vi "Test Zentral Trigger PC.vi"() -> ()   [LabVIEW 2009]
uses:
  LV-BME Interface/ChnlSettings.ctl
  LV-BME Interface/BME_DG_TriggerSettings.ctl
  DG Classes/BME_DG_G05P2/SG05P2 Clock and Trigger Settings.ctl
  LV-BME Interface/ClockSource.ctl
  DG Classes/BME_DG_System/BME_DG_System.lvclass
  DG Classes/BME_DG_G05P2/BME_DG_G05P2.lvclass
  DG Classes/BME_DG_G05P2_Chnl/BME_DG_G05P2_Chnl.lvclass
  ChnlParam.ctl
  DG Classes/BME_DG_Base/BME_DG_Base.lvclass
  DG Classes/BME_DG_Chnl/BME_DG_Chnl.lvclass
panel:
  in  "Karten Parameter":T1[](array[typedef])=[{"Trigger"={"InputTerminated?"=TRUE, "InternalClockPeriode(µs)"=0.106293, "TriggerLevel"=-0.1001, "PresetValue"=0, "DivideBy"=4, "Clock Source"=3, "Gate Divider"=1, "PositiveGate?"=TRUE, "InternalTrigger?"=TRUE, "InternalArm?"=FALSE, "SWTrigger?"=FALSE, "RisingEdge?"=FALSE, "StopOnPreset?"=FALSE, "ResetWhenDone?"=FALSE, "TriggerEnabled?"=TRUE}, "ClockSource "=3, "V2 Trigger"={"Gate Type"=TRUE, "Synchronize Gate"=FALSE, "Force Trigger (µs)"=0.0, "MS Bus"=24}, " crystal oscillator"=6, "CardName"="Mira Sync"}, {"Trigger"={"InputTerminated?"=TRUE, "InternalClockPeriode(µs)"=99999.989371, "TriggerLevel"=1.401, "PresetValue"=0, "DivideBy"=1, "Clock Source"=3, "Gate Divider"=1, "PositiveGate?"=TRUE, "InternalTrigger?"=TRUE, "InternalArm?"=FALSE, "SWTrigger?"=FALSE, "RisingEdge?"=FALSE, "StopOnPreset?"=FALSE, "ResetWhenDone?"=FALSE, "TriggerEnabled?"=TRUE}, "ClockSource "=2, "V2 Trigger"={"Gate Type"=TRUE, "Synchronize Gate"=FALSE, "Force Trigger (µs)"=0.0, "MS Bus"=24}, " crystal oscillator"=1, "CardName"="FE PP"}, {"Trigger"={"InputTerminated?"=FALSE, "InternalClockPeriode(µs)"=0.0, "TriggerLevel"=1.25, "PresetValue"=0, "DivideBy"=1, "Clock Source"=3, "Gate Divider"=1, "PositiveGate?"=TRUE, "InternalTrigger?"=FALSE, "InternalArm?"=FALSE, "SWTrigger?"=FALSE, "RisingEdge?"=FALSE, "StopOnPreset?"=FALSE, "ResetWhenDone?"=FALSE, "TriggerEnabled?"=TRUE}, "ClockSource "=4, "V2 Trigger"={"Gate Type"=TRUE, "Synchronize Gate"=FALSE, "Force Trigger (µs)"=0.0, "MS Bus"=16}, " crystal oscillator"=8, "CardName"="A1 Haupt"}, {"Trigger"={"InputTerminated?"=TRUE, "InternalClockPeriode(µs)"=0.0, "TriggerLevel"=1.25, "PresetValue"=0, "DivideBy"=1, "Clock Source"=3, "Gate Divider"=1, "PositiveGate?"=TRUE, "InternalTrigger?"=FALSE, "InternalArm?"=FALSE, "SWTrigger?"=FALSE, "RisingEdge?"=FALSE, "StopOnPreset?"=FALSE, "ResetWhenDone?"=FALSE, "TriggerEnabled?"=TRUE}, "ClockSource "=4, "V2 Trigger"={"Gate Type"=TRUE, "Synchronize Gate"=FALSE, "Force Trigger (µs)"=0.0, "MS Bus"=16}, " crystal oscillator"=8, "CardName"="A1 Neben"}, {"Trigger"={"InputTerminated?"=FALSE, "InternalClockPeriode(µs)"=0.0, "TriggerLevel"=1.25, "PresetValue"=0, "DivideBy"=1, "Clock Source"=3, "Gate Divider"=1, "PositiveGate?"=TRUE, "InternalTrigger?"=TRUE, "InternalArm?"=FALSE, "SWTrigger?"=FALSE, "RisingEdge?"=FALSE, "StopOnPreset?"=FALSE, "ResetWhenDone?"=FALSE, "TriggerEnabled?"=TRUE}, "ClockSource "=4, "V2 Trigger"={"Gate Type"=TRUE, "Synchronize Gate"=FALSE, "Force Trigger (µs)"=0.0, "MS Bus"=16}, " crystal oscillator"=8, "CardName"="A2 Haupt"}, {"Trigger"={"InputTerminated?"=TRUE, "InternalClockPeriode(µs)"=0.0, "TriggerLevel"=1.25, "PresetValue"=0, "DivideBy"=1, "Clock Source"=3, "Gate Divider"=1, "PositiveGate?"=TRUE, "InternalTrigger?"=FALSE, "InternalArm?"=FALSE, "SWTrigger?"=FALSE, "RisingEdge?"=FALSE, "StopOnPreset?"=FALSE, "ResetWhenDone?"=FALSE, "TriggerEnabled?"=TRUE}, "ClockSource "=4, "V2 Trigger"={"Gate Type"=TRUE, "Synchronize Gate"=FALSE, "Force Trigger (µs)"=0.0, "MS Bus"=16}, " crystal oscillator"=1, "CardName"="A2 Neben"}, {"Trigger"={"InputTerminated?"=TRUE, "InternalClockPeriode(µs)"=0.0, "TriggerLevel"=1.25, "PresetValue"=0, "DivideBy"=1, "Clock Source"=3, "Gate Divider"=1, "PositiveGate?"=TRUE, "InternalTrigger?"=FALSE, "InternalArm?"=FALSE, "SWTrigger?"=FALSE, "RisingEdge?"=FALSE, "StopOnPreset?"=FALSE, "ResetWhenDone?"=FALSE, "TriggerEnabled?"=TRUE}, "ClockSource "=4, "V2 Trigger"={"Gate Type"=TRUE, "Synchronize Gate"=FALSE, "Force Trigger (µs)"=0.0, "MS Bus"=16}, " crystal oscillator"=1, "CardName"="A2 PP"}, {"Trigger"={"InputTerminated?"=TRUE, "InternalClockPeriode(µs)"=0.0, "TriggerLevel"=1.25, "PresetValue"=0, "DivideBy"=1, "Clock Source"=3, "Gate Divider"=1, "PositiveGate?"=TRUE, "InternalTrigger?"=FALSE, "InternalArm?"=FALSE, "SWTrigger?"=FALSE, "RisingEdge?"=FALSE, "StopOnPreset?"=FALSE, "ResetWhenDone?"=FALSE, "TriggerEnabled?"=TRUE}, "ClockSource "=4, "V2 Trigger"={"Gate Type"=TRUE, "Synchronize Gate"=FALSE, "Force Trigger (µs)"=0.0, "MS Bus"=16}, " crystal oscillator"=1, "CardName"="A2 PP, A2.5"}, {"Trigger"={"InputTerminated?"=TRUE, "InternalClockPeriode(µs)"=0.0, "TriggerLevel"=1.25, "PresetValue"=0, "DivideBy"=1, "Clock Source"=3, "Gate Divider"=1, "PositiveGate?"=TRUE, "InternalTrigger?"=FALSE, "InternalArm?"=FALSE, "SWTrigger?"=FALSE, "RisingEdge?"=FALSE, "StopOnPreset?"=FALSE, "ResetWhenDone?"=FALSE, "TriggerEnabled?"=TRUE}, "ClockSource "=4, "V2 Trigger"={"Gate Type"=TRUE, "Synchronize Gate"=FALSE, "Force Trigger (µs)"=0.0, "MS Bus"=16}, " crystal oscillator"=1, "CardName"="A3 Haupt"}, {"Trigger"={"InputTerminated?"=TRUE, "InternalClockPeriode(µs)"=0.0, "TriggerLevel"=1.25, "PresetValue"=0, "DivideBy"=1, "Clock Source"=3, "Gate Divider"=1, "PositiveGate?"=TRUE, "InternalTrigger?"=FALSE, "InternalArm?"=FALSE, "SWTrigger?"=FALSE, "RisingEdge?"=FALSE, "StopOnPreset?"=FALSE, "ResetWhenDone?"=FALSE, "TriggerEnabled?"=TRUE}, "ClockSource "=4, "V2 Trigger"={"Gate Type"=TRUE, "Synchronize Gate"=FALSE, "Force Trigger (µs)"=0.0, "MS Bus"=16}, " crystal oscillator"=1, "CardName"="A4 Haupt"}] {"V2 Trigger"."MS Bus" format="%04x" items=["Local Primary"=1, "Local Secondary"=2, "Local Force"=4, "Resynchronize"=8, "Master Primary"=16, "Master Secondary"=32, "Master Force"=64, "System Clock"=128, "Delay Clock"=256, "Inhibit Local"=512, "Start Local"=1024, "Start Bus"=2048, "Step Back Local"=4096, "Step Back Bus"=8192, "Enable From E"=65536, "Enable From F"=131072, "Enable From Bus"=262144]; "V2 Trigger"."Force Trigger (µs)" min=0.0 format="%.6f"; "ClockSource" items=["Internal Oscillator"=1, "External Trigger"=2, "Trigger & Oscillator"=3, "MasterSlave Bus"=4]; "Trigger"."Gate Divider" min=1 max=1000000; "Trigger"."Clock Source" items=["Internal Oscillator"=1, "External Trigger"=2, "Trigger & Oscillator"=3]; "Trigger"."InternalClockPeriode(µs)" format="%#_11g"}
  in  "Go Signal":u32(ring)=2048 items=["Local Primary"=1, "Local Secondary"=2, "Local Force"=4, "Resynchronize"=8, "Master Primary"=16, "Master Secondary"=32, "Master Force"=64, "System Clock"=128, "Delay Clock"=256, "Inhibit Local"=512, "Start Local"=1024, "Start Bus"=2048, "Step Back Local"=4096, "Step Back Bus"=8192, "From E"=65536, "From F"=131072, "From Bus"=262144]
  out "Problem Chnls out":string[](array[string])
  out "DelayFormulas":string[](array[string])
  in  "Reset Error":bool
  out "error out":errorcluster
  in  "Update Delay formula":bool=TRUE
  in  "DelayFormula":string="MasterSG02P2_ChnlT0 + 100"
  in  "Aknowledge interrupts":bool
  in  "stop 3":bool=TRUE
  in  "SetDelay":bool=TRUE
  in  "UpdateChnl":bool=TRUE
  in  "ChnlParameter":T5 {"ChnParam2write"."Delay (µs)" min=0.0 max=100000000.0 format="%.5f"}
  out "CountsRemains":i32
  out "TriggerCounters":i32[](array[numeric])
  out "Interrupts":u32[](array[numeric]) format="%b"
  out "RemainingTriggers":T6(array[cluster])=[[{"Time Stamp"=timestamp(3416308194.6875 s since 1904-01-01), "Numeric"=-64}, {"Time Stamp"=timestamp(3416308194.6875 s since 1904-01-01), "Numeric"=4}, {"Time Stamp"=timestamp(3416308194.6875 s since 1904-01-01), "Numeric"=-64}, {"Time Stamp"=timestamp(3416308194.6875 s since 1904-01-01), "Numeric"=-64}], [{"Time Stamp"=timestamp(3416308194.6875 s since 1904-01-01), "Numeric"=-64}, {"Time Stamp"=timestamp(3416308194.6875 s since 1904-01-01), "Numeric"=-64}, {"Time Stamp"=timestamp(3416308194.6875 s since 1904-01-01), "Numeric"=-64}, {"Time Stamp"=timestamp(3416308194.6875 s since 1904-01-01), "Numeric"=-64}], [{"Time Stamp"=timestamp(3416308194.6875 s since 1904-01-01), "Numeric"=-64}, {"Time Stamp"=timestamp(3416308194.6875 s since 1904-01-01), "Numeric"=-64}, {"Time Stamp"=timestamp(3416308194.6875 s since 1904-01-01), "Numeric"=-64}, {"Time Stamp"=timestamp(3416308194.6875 s since 1904-01-01), "Numeric"=-64}]] {"Time Stamp" format="%<%I:%M:%S%3u %p>T"}
  in  "stop 2":bool=TRUE
  in  "ReadStatus":bool=TRUE
  in  "Activate":bool
  in  "ResetModuloCounters":bool=TRUE
  in  "TriggerModulo":u32=4
  out "Modulo Settings":u32[](array[numeric])
  out "Chnls":T4[](array[typedef])=[{" Delay (µs)"=0.0, "On? (false)"=TRUE, "PositiveVoltage?"=TRUE, "50OhmTerminated? "=TRUE, "25OhmOutput?"=FALSE}, {" Delay (µs)"=0.0, "On? (false)"=TRUE, "PositiveVoltage?"=TRUE, "50OhmTerminated? "=TRUE, "25OhmOutput?"=FALSE}, {" Delay (µs)"=0.0, "On? (false)"=TRUE, "PositiveVoltage?"=TRUE, "50OhmTerminated? "=TRUE, "25OhmOutput?"=FALSE}] {"Delay (µs)" min=0.0 max=100000000.0 format="%.5f"}
  in  "Trigger Base":T2={"InputTerminated?"=FALSE, "InternalClockPeriode(µs)"=1000000.0, "TriggerLevel"=1.25, "PresetValue"=0, "DivideBy"=1, "Clock Source"=1, "Gate Divider"=1, "PositiveGate?"=TRUE, "InternalTrigger?"=FALSE, "InternalArm?"=FALSE, "SWTrigger?"=FALSE, "RisingEdge?"=FALSE, "StopOnPreset?"=FALSE, "ResetWhenDone?"=TRUE, "TriggerEnabled?"=TRUE} {"Gate Divider" min=1 max=1000000; "Clock Source" items=["Internal Oscillator"=1, "External Trigger"=2, "Trigger & Oscillator"=3]; "InternalClockPeriode(µs)" format="%#_11g"}
  in  "Selected Chnl":u16(ring) items=["MasterSG02P2_ChnlT0", "MasterSG02P2_ChnlA", "MasterSG02P2_ChnlB"]
  in  "Selected Card":u16(ring)=1 items=["MasterSG02P2", "Slave 1", "Slave 2", "MasterS08P1"]
  in  "STOP":bool=TRUE
  in  "ChnParam2write":T4={" Delay (µs)"=0.0, "On? (false)"=TRUE, "PositiveVoltage?"=TRUE, "50OhmTerminated? "=TRUE, "25OhmOutput?"=FALSE} {"Delay (µs)" min=0.0 max=100000000.0 format="%.5f"}
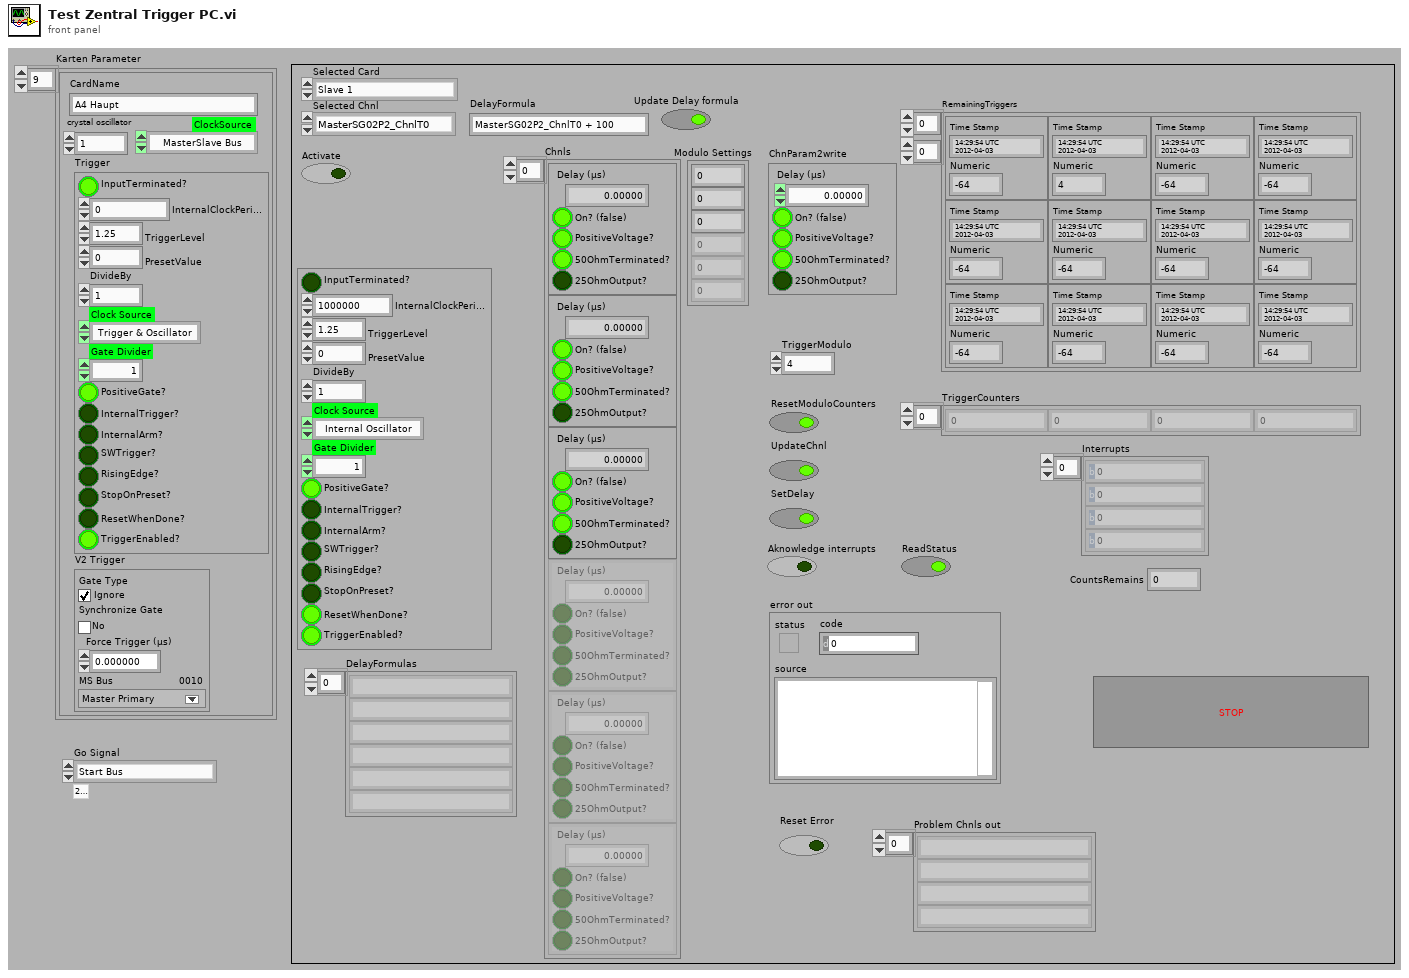
[diagram p1: front panel]
types:
  T1 = typedef "SG05P2 Clock and Trigger Settings.ctl" = cluster{"Trigger":T2, "ClockSource ":T3, "V2 Trigger":cluster{"Gate Type":bool, "Synchronize Gate":bool, "Force Trigger (µs)":dbl, "MS Bus":u32}, " crystal oscillator":u32, "CardName":string}
  T2 = typedef "BME_DG_TriggerSettings.ctl" = cluster{"InputTerminated?":bool, "InternalClockPeriode(µs)":dbl, "TriggerLevel":dbl, "PresetValue":i32, "DivideBy":i32, "Clock Source":u32, "Gate Divider":i32, "PositiveGate?":bool, "InternalTrigger?":bool, "InternalArm?":bool, "SWTrigger?":bool, "RisingEdge?":bool, "StopOnPreset?":bool, "ResetWhenDone?":bool, "TriggerEnabled?":bool}
  T3 = typedef "ClockSource.ctl" = i32
  T4 = typedef "ChnlSettings.ctl" = cluster{" Delay (µs)":dbl, "On? (false)":bool, "PositiveVoltage?":bool, "50OhmTerminated? ":bool, "25OhmOutput?":bool}
  T5 = cluster{"ChnlName":string, "ChnParam2write":T4, "TriggerModulo":u32}
  T6 = cluster{"Time Stamp":timestamp, "Numeric":i32}[][]
  T7 = typedef "ChnlParam.ctl" = cluster{"ChnlName":string, "DelayFormula":string, "OutputModulo":i32}
  T8 = cluster{"Gate Type":bool, "Synchronize Gate":bool, "Force Trigger (µs)":dbl, "MS Bus":u32}
  T9 = enum8{"Enabled", "Disabled", "Disabled and Grayed Out"}
  T10 = cluster{"ChnlName":string, "ChnParam2write":T4, "TriggerModulo":u32}[]
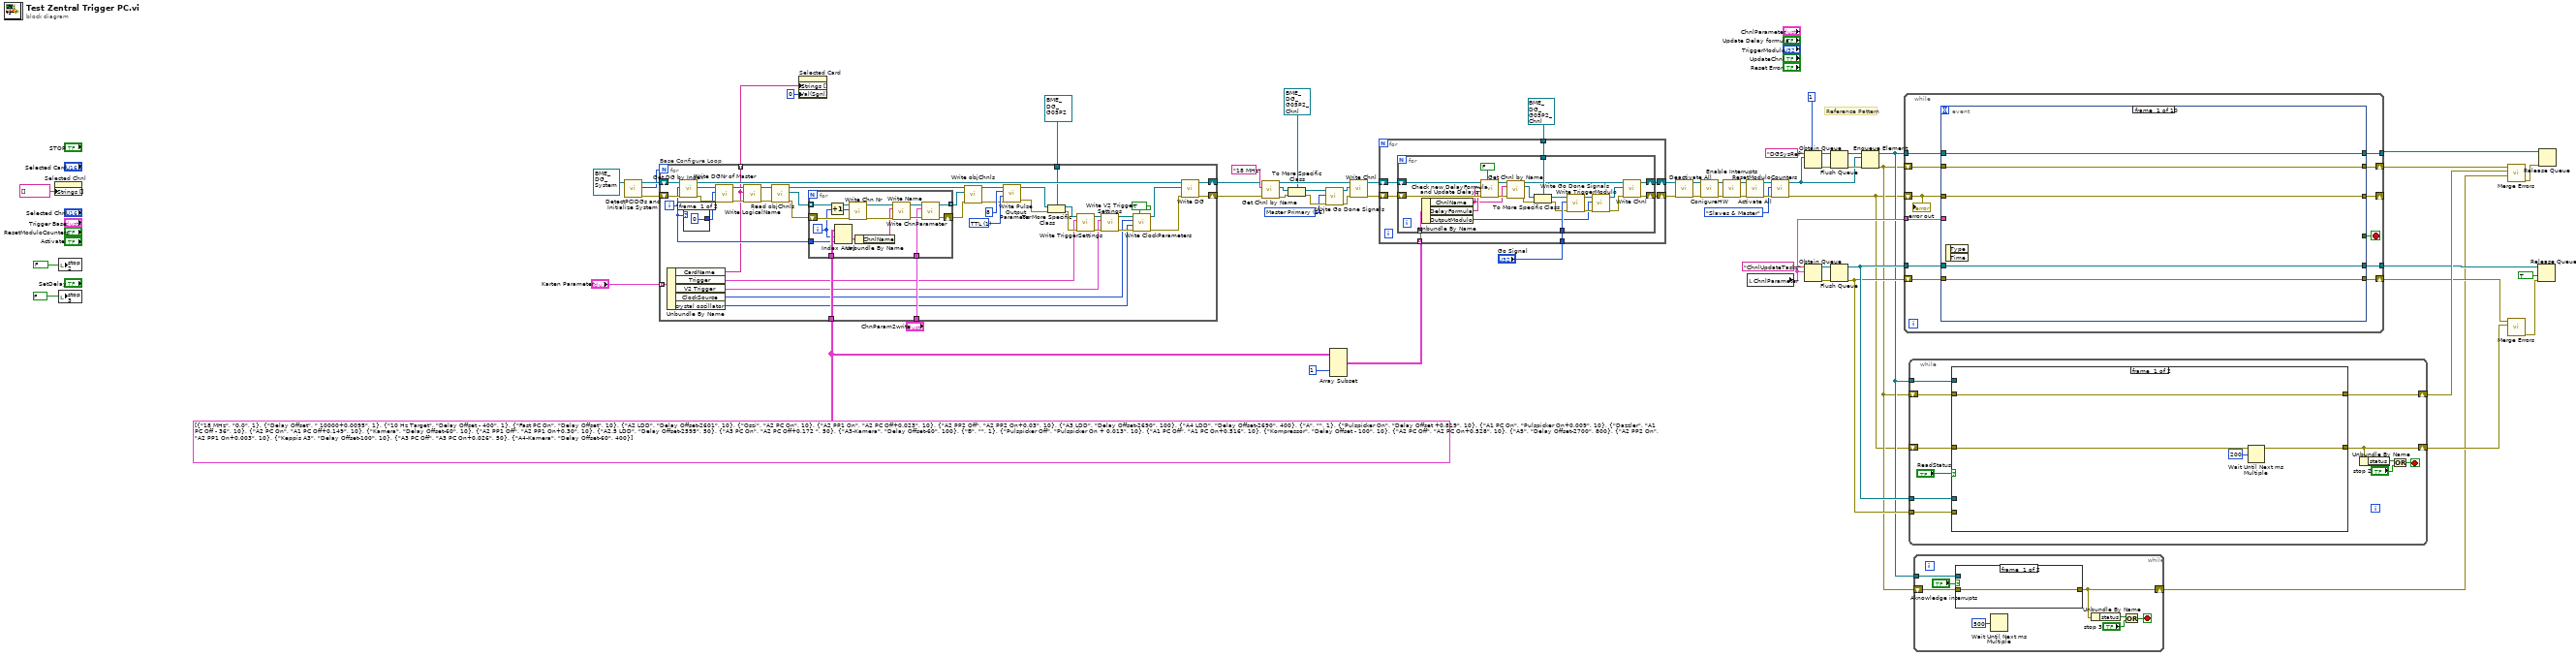
[diagram p0: block diagram]
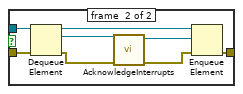
[diagram p2: hidden frame]
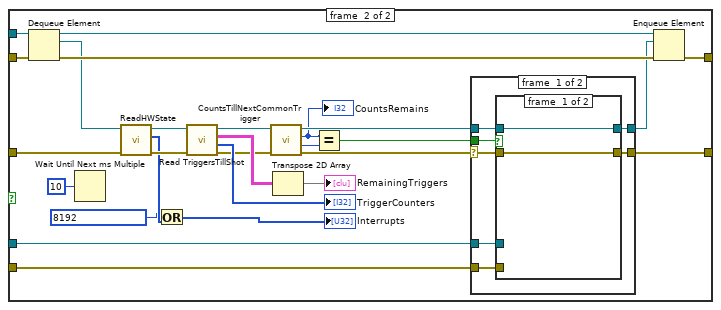
[diagram p3: hidden frame]
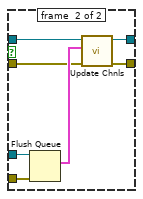
[diagram p4: hidden frame]
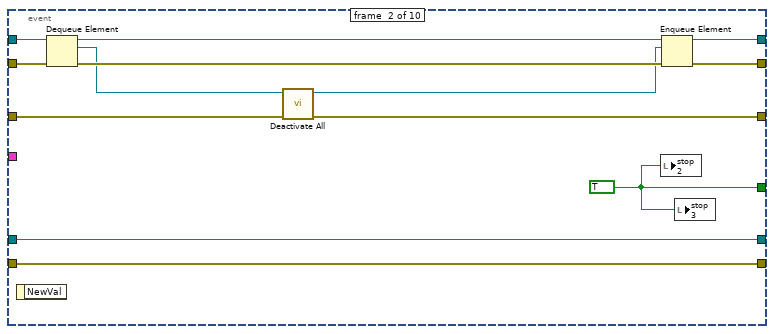
[diagram p6: hidden frame]
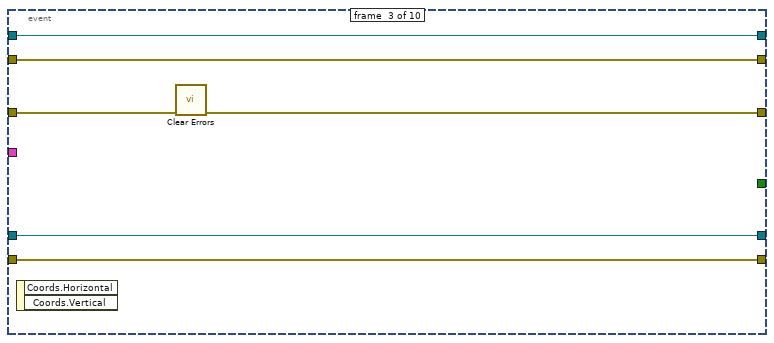
[diagram p7: hidden frame]
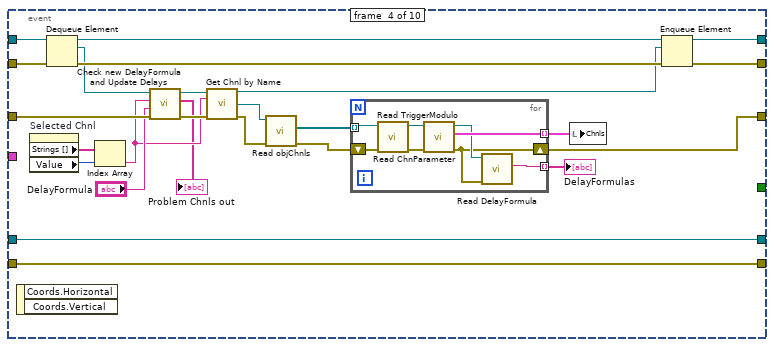
[diagram p8: hidden frame]
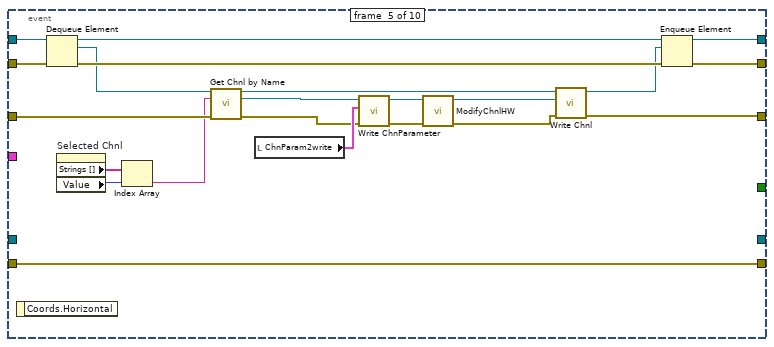
[diagram p9: hidden frame]
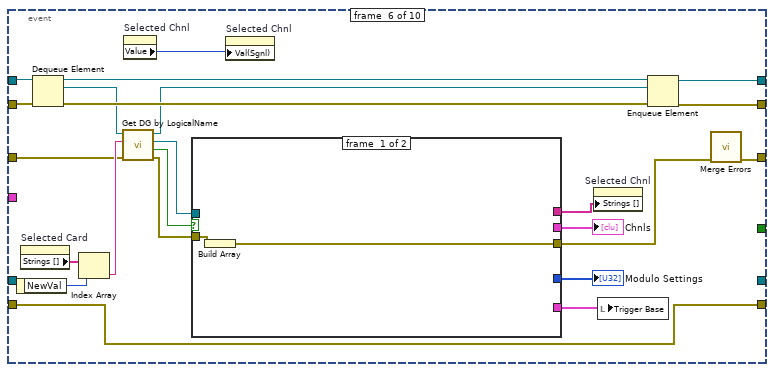
[diagram p10: hidden frame]
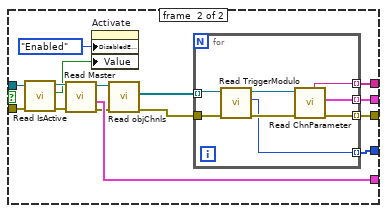
[diagram p11: hidden frame]
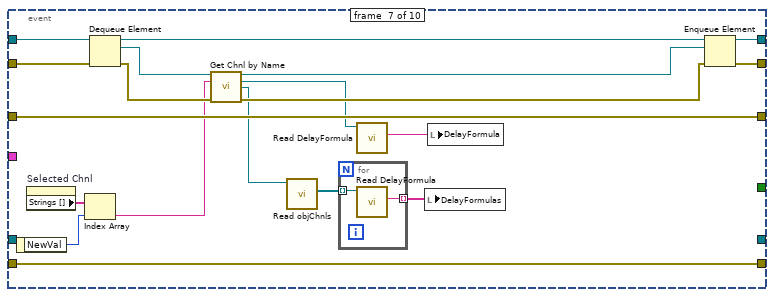
[diagram p12: hidden frame]
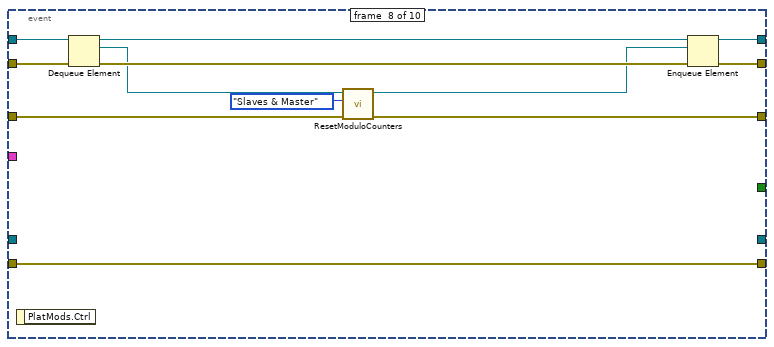
[diagram p13: hidden frame]
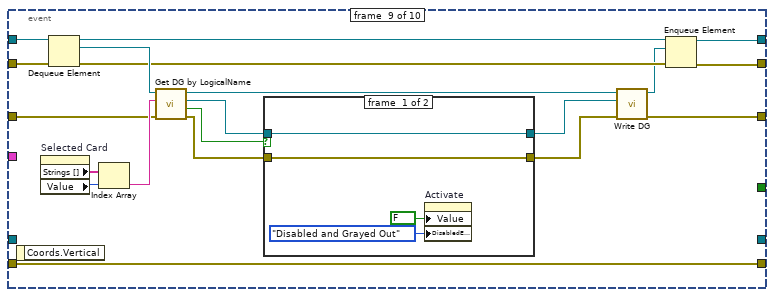
[diagram p14: hidden frame]
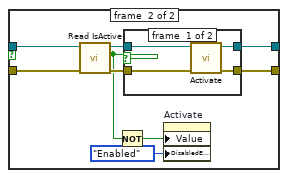
[diagram p15: hidden frame]
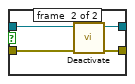
[diagram p16: hidden frame]
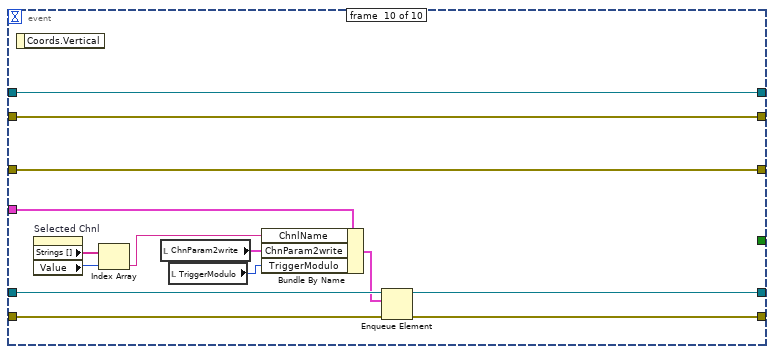
[diagram p17: hidden frame]
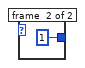
[diagram p18: hidden frame]
diagram:
  w10 = T7[][] [[{"ChnlName"="18 MHz", "DelayFormula"="0.0", "OutputModulo"=1}, {"ChnlName"="Delay Offset", "DelayFormula"=" 10000+0.0095", "OutputModulo"=1}, {"ChnlName"="10 Hz Target", "DelayFormula"="Delay Offset - 400", "OutputModulo"=1}, {"ChnlName"="Fast PC On", "DelayFormula"="Delay Offset", "OutputModulo"=10}, {"ChnlName"="A2 LDD", "DelayFormula"="Delay Offset-2601", "OutputModulo"=10}, {"ChnlName"="Oszi", "DelayFormula"="A2 PC On", "OutputModulo"=10}, {"ChnlName"="A2 PP1 On", "DelayFormula"="A2 PC Off+0.023", "OutputModulo"=10}, {"ChnlName"="A2 PP2 Off", "DelayFormula"="A2 PP2 On+0.03", "OutputModulo"=10}, {"ChnlName"="A3 LDD", "DelayFormula"="Delay Offset-2690", "OutputModulo"=100}, {"ChnlName"="A4 LDD", "DelayFormula"="Delay Offset-2690", "OutputModulo"=400}], [{"ChnlName"="A", "DelayFormula"="", "OutputModulo"=1}, {"ChnlName"="Pulspicker On", "DelayFormula"="Delay Offset +0.819", "OutputModulo"=10}, {"ChnlName"="A1 PC On", "DelayFormula"="Pulspicker On+0.009", "OutputModulo"=10}, {"ChnlName"="Dazzler", "DelayFormula"="A1 PC Off - 36", "OutputModulo"=10}, {"ChnlName"="A2 PC On", "DelayFormula"="A1 PC Off+0.149", "OutputModulo"=10}, {"ChnlName"="Kamera", "DelayFormula"="Delay Offset-60", "OutputModulo"=10}, {"ChnlName"="A2 PP1 Off", "DelayFormula"="A2 PP1 On+0.30", "OutputModulo"=10}, {"ChnlName"="A2.5 LDD", "DelayFormula"="Delay Offset-2595", "OutputModulo"=50}, {"ChnlName"="A3 PC On", "DelayFormula"="A2 PC Off+0.172 ", "OutputModulo"=50}, {"ChnlName"="A3-Kamera", "DelayFormula"="Delay Offset-60", "OutputModulo"=100}], [{"ChnlName"="B", "DelayFormula"="", "OutputModulo"=1}, {"ChnlName"="Pulspicker Off", "DelayFormula"="Pulspicker On + 0.013", "OutputModulo"=10}, {"ChnlName"="A1 PC Off", "DelayFormula"="A1 PC On+0.516", "OutputModulo"=10}, {"ChnlName"="Kompressor", "DelayFormula"="Delay Offset - 100", "OutputModulo"=10}, {"ChnlName"="A2 PC Off", "DelayFormula"="A2 PC On+0.528", "OutputModulo"=10}, {"ChnlName"="A5", "DelayFormula"="Delay Offset-2700", "OutputModulo"=800}, {"ChnlName"="A2 PP2 On", "DelayFormula"="A2 PP1 On+0.003", "OutputModulo"=10}, {"ChnlName"="Keppis A3", "DelayFormula"="Delay Offset-100", "OutputModulo"=10}, {"ChnlName"="A3 PC Off", "DelayFormula"="A3 PC On+0.026", "OutputModulo"=50}, {"ChnlName"="A4-Kamera", "DelayFormula"="Delay Offset-60", "OutputModulo"=400}]] ("ChnlParam 2")
  w14 = u32 16 items=["Local Primary"=1, "Local Secondary"=2, "Local Force"=4, "Resynchronize"=8, "Master Primary"=16, "Master Secondary"=32, "Master Force"=64, "System Clock"=128, "Delay Clock"=256, "Inhibit Local"=512, "Start Local"=1024, "Start Bus"=2048, "Step Back Local"=4096, "Step Back Bus"=8192, "From E"=65536, "From F"=131072, "From Bus"=262144] ("Go Signal")
  # "Reference Pattern"
  n1 = property on="Selected Chnl" class="Ring (strict)"("Strings []"=string[] []) -> ()  [unwired: 2 in, 2 out]
  n2 = local write "stop 2"(FALSE ("stop 2")) -> ()
  n3 = local write "stop 3"(FALSE ("stop 3")) -> ()
  n4 = call "DetectPCIDGs and Initialize System.vi"("BME_DG_System in"=refnum<class "BME_DG_System.lvclass"> refnum ("BME_DG_System.lvclass")) -> ("error out"=w66:errorcluster, "NumberOfCards"=w65:i32, "BME_DG_System out"=w67:refnum<class "BME_DG_System.lvclass">)  [unwired: 8 in]
  n5 = for "Base Configure Loop" {
    N: w65 -> [_]
    shift-right: [w107] -> w5
    shift-left: w67 -> [w110]
    shift-right: [w106] -> w4
    shift-left: w66 -> [w109]
    tunnel: "ChnParam2write" -> [w103]
    tunnel: w10 -> [w99]
    tunnel: [w85] -> w39 mode=indexing
    tunnel: "Karten Parameter" -> [w86] mode=indexing
    tunnel: refnum<class "BME_DG_G05P2.lvclass"> refnum ("BME_DG_G05P2.lvclass") -> [w78]
    i -> [w92]
    w88 = u32 1 items=["TTL"=1, "NIM"=2, "ECL"=3] ("Pulse Output Level")
    n6 = Unbundle By Name(w86) -> ("CardName"=w85:string, "Trigger"=w72:T2, "V2 Trigger"=w71:T8, "ClockSource"=w69:T3, "crystal oscillator"=w70:u32)
    n7 = call "Get DG by Index.vi"("error in (no error)"=w109, "index"=w92, "BME_DG_System in"=w110) -> ("error out"=w93:errorcluster, "BME_DG_Base.lvclass"=w96:refnum<class "BME_DG_Base.lvclass">, "BME_DG_System out"=w108:refnum<class "BME_DG_System.lvclass">)  [unwired: 6 in]
    n8 = case shown="1, Default" w92 {
      tunnel: [0 1] -> w91
      frame #0 {
      }
      frame #1 {
      }
    }
    n9 = call-dynamic "Write DGNr of Master.vi"("error in (no error)"=w93, "DGNr of Master"=w91, "BME_DG_Base in"=w96) -> ("error out"=w94:errorcluster, "BME_DG_Base out"=w95:refnum<class "BME_DG_Base.lvclass">)  [unwired: 7 in]
    n10 = call "Write LogicalName.vi"("error in (no error)"=w94, "LogicalName"=w85, "BME_DG_Base in"=w95) -> ("error out"=w97:errorcluster, "BME_DG_Base out"=w98:refnum<class "BME_DG_Base.lvclass">)  [unwired: 7 in]
    n11 = call-dynamic "Read objChnls.vi"("error in (no error)"=w97, "BME_DG_Base in"=w98) -> ("error out"=w104:errorcluster, "objChnls"=w105:refnum<class "BME_DG_Chnl.lvclass">[], "BME_DG_Base out"=w101:refnum<class "BME_DG_Base.lvclass">)  [unwired: 6 in, 1 out]
    n12 = for {
      tunnel: w105 -> [w124] mode=indexing
      shift-right: [w116] -> w100
      shift-left: w104 -> [w122]
      tunnel: w103 -> [w125]
      tunnel: [w117] -> w102 mode=indexing
      tunnel: w99 -> [w119]
      tunnel: w92 -> [w114]
      i -> [w115]
      n13 = Increment(x=w115) -> (x+1=w120:i32)
      n14 = Index Array(array=w119, index (row)=w115, index (col)=w114) -> (element=w118:T7)
      n15 = call-dynamic "Write Chn Nr.vi"("error in (no error)"=w122, "Chn Nr"=w120, "BME_DG_Chnl in"=w124) -> ("error out"=w121:errorcluster, "BME_DG_Chnl out"=w123:refnum<class "BME_DG_Chnl.lvclass">)  [unwired: 7 in]
      n16 = Unbundle By Name(w118) -> ("ChnlName"=w113:string)
      n17 = call-dynamic "Write Name.vi"("error in (no error)"=w121, "Name"=w113, "BME_DG_Chnl in"=w123) -> ("error out"=w126:errorcluster, "BME_DG_Chnl out"=w127:refnum<class "BME_DG_Chnl.lvclass">)  [unwired: 7 in]
      n18 = call-dynamic "Write ChnParameter.vi"("error in (no error)"=w126, "ChnParemater"=w125, "BME_DG_Chnl in"=w127) -> ("error out"=w116:errorcluster, "BME_DG_Chnl out"=w117:refnum<class "BME_DG_Chnl.lvclass">)  [unwired: 7 in]
    }
    n19 = call-dynamic "Write objChnls.vi"("error in (no error)"=w100, "objChnls"=w102, "BME_DG_Base in"=w101) -> ("error out"=w87:errorcluster, "BME_DG_Base out"=w90:refnum<class "BME_DG_Base.lvclass">)  [unwired: 7 in]
    n20 = call-dynamic "Write Pulse Output Parameter.vi"("error in (no error)"=w87, "Pulse Output Level"=w88, "Pulse Width"=u32 8, "BME_DG_Base in"=w90) -> ("error out"=w75:errorcluster, "BME_DG_Base out"=w77:refnum<class "BME_DG_Base.lvclass">)  [unwired: 6 in]
    n21 = To More Specific Class(target class=w78, reference=w77, error in=w75) -> (specific class reference=w79:refnum<class "BME_DG_G05P2.lvclass">, error out=w80:errorcluster)
    n22 = call-dynamic "Write TriggerSettings.vi"("error in (no error)"=w80, "Trigger Settings"=w72, "BME_DG_Base in"=w79) -> ("error out"=w83:errorcluster, "BME_DG_Base out"=w81:refnum<class "BME_DG_G05P2.lvclass">)  [unwired: 7 in]
    n23 = call-dynamic "Write V2 Trigger Settings.vi"("error in (no error)"=w83, "V2 Trigger Settings"=w71, "BME_DG_G05 in"=w81) -> ("error out"=w84:errorcluster, "BME_DG_G05 out"=w82:refnum<class "BME_DG_G05P2.lvclass">)  [unwired: 7 in]
    n24 = call-dynamic "Write ClockParameters.vi"("ClockEnable"=TRUE, "error in (no error)"=w84, "PrescalerCrystalOscilator"=w70, "ClockSource"=w69, "BME_DG_Base in"=w82) -> ("error out"=w74:errorcluster, "BME_DG_Base out"=w76:refnum<class "BME_DG_G05P2.lvclass">)  [unwired: 5 in]
    n25 = call "Write DG.vi"("error in (no error)"=w74, "BME_DG_Base"=w76, "BME_DG_System in"=w108) -> ("error out"=w106:errorcluster, "BME_DG_System out"=w107:refnum<class "BME_DG_System.lvclass">)  [unwired: 7 in]
  }
  n26 = property on="Selected Card" class="Ring (strict)"("Strings []"=w39, "Val(Sgnl)"=u16 0 ("Value (Signaling)")) -> ()  [unwired: 2 in, 2 out]
  n27 = call "Get Chnl by Name.vi"("BME_DG_System in"=w5, "Chnl Name"="18 MHz", "error in (no error)"=w4) -> ("BME_DG_System out"=w22:refnum<class "BME_DG_System.lvclass">, "BME_DG_Chnl"=w21:refnum<class "BME_DG_Chnl.lvclass">, "error out"=w18:errorcluster)  [unwired: 7 in, 3 out]
  n28 = To More Specific Class(target class=refnum<class "BME_DG_G05P2_Chnl.lvclass"> refnum ("BME_DG_G05P2_Chnl.lvclass"), reference=w21, error in=w18) -> (specific class reference=w20:refnum<class "BME_DG_G05P2_Chnl.lvclass">, error out=w17:errorcluster)
  n29 = call-dynamic "Write Go Done Signals.vi"("error in (no error)"=w17, "Go Signal"=w14, "BME_DG_G05P2_Chnl in"=w20) -> ("error out"=w16:errorcluster, "BME_DG_G05P2_Chnl out"=w15:refnum<class "BME_DG_G05P2_Chnl.lvclass">)  [unwired: 7 in]
  n30 = Array Subset(array=w10, index (col)=1 ("index")) -> (w11:T7[][])  [unwired: 3 in]
  n31 = call "Write Chnl.vi"("error in (no error)"=w16, "BME_DG_Chnl.lvclass"=w15, "BME_DG_System in"=w22) -> ("error out"=w1:errorcluster, "BME_DG_System out"=w2:refnum<class "BME_DG_System.lvclass">)  [unwired: 7 in]
  n32 = for {
    shift-right: [w133] -> w13
    shift-left: w2 -> [w134]
    shift-right: [w131] -> w12
    shift-left: w1 -> [w132]
    tunnel: w11 -> [w130] mode=indexing
    tunnel: refnum<class "BME_DG_G05P2_Chnl.lvclass"> refnum ("BME_DG_G05P2_Chnl.lvclass") -> [w129]
    tunnel: "Go Signal" -> [w128]
    n33 = for {
      shift-right: [w139] -> w133
      shift-left: w134 -> [w156]
      shift-right: [w138] -> w131
      shift-left: w132 -> [w155]
      tunnel: w130 -> [w153] mode=indexing
      tunnel: w129 -> [w147]
      tunnel: w128 -> [w145]
      n34 = Unbundle By Name(w153) -> ("ChnlName"=w149:string, "DelayFormula"=w152:string, "OutputModulo"=w140:i32)
      n35 = call "Check new DelayFormula and Update Delays.vi"("Update HW"=FALSE, "error in (no error)"=w155, "Delay Formula"=w152, "ChnlName"=w149, "BME_DG_System in"=w156) -> ("error out"=w150:errorcluster, "BME_DG_System out"=w151:refnum<class "BME_DG_System.lvclass">)  [unwired: 4 in, 1 out]
      n36 = call "Get Chnl by Name.vi"("BME_DG_System in"=w151, "Chnl Name"=w149, "error in (no error)"=w150) -> ("BME_DG_System out"=w137:refnum<class "BME_DG_System.lvclass">, "BME_DG_Chnl"=w146:refnum<class "BME_DG_Chnl.lvclass">, "error out"=w144:errorcluster)  [unwired: 7 in, 3 out]
      n37 = To More Specific Class(target class=w147, reference=w146, error in=w144) -> (specific class reference=w148:refnum<class "BME_DG_G05P2_Chnl.lvclass">, error out=w143:errorcluster)
      n38 = call-dynamic "Write Go Done Signals.vi"("error in (no error)"=w143, "Go Signal"=w145, "BME_DG_G05P2_Chnl in"=w148) -> ("error out"=w141:errorcluster, "BME_DG_G05P2_Chnl out"=w142:refnum<class "BME_DG_G05P2_Chnl.lvclass">)  [unwired: 7 in]
      n39 = call-dynamic "Write TriggerModulo.vi"("error in (no error)"=w141, "TriggerModulo"=w140, "BME_DG_G05_Chnl in"=w142) -> ("error out"=w136:errorcluster, "BME_DG_G05_Chnl out"=w135:refnum<class "BME_DG_G05P2_Chnl.lvclass">)  [unwired: 7 in]
      n40 = call "Write Chnl.vi"("error in (no error)"=w136, "BME_DG_Chnl.lvclass"=w135, "BME_DG_System in"=w137) -> ("error out"=w138:errorcluster, "BME_DG_System out"=w139:refnum<class "BME_DG_System.lvclass">)  [unwired: 7 in]
    }
  }
  n41 = call "Deactivate All.vi"("error in (no error)"=w12, "BME_DG_System in"=w13) -> ("error out"=w37:errorcluster, "BME_DG_System out"=w38:refnum<class "BME_DG_System.lvclass">)  [unwired: 8 in]
  n42 = call "ConigureHW.vi"("error in (no error)"=w37, "BME_DG_System in"=w38) -> ("error out"=w35:errorcluster, "BME_DG_System out"=w36:refnum<class "BME_DG_System.lvclass">)  [unwired: 8 in]
  n43 = call "Enable Interrupts.vi"("error in (no error)"=w35, "BME_DG_System in"=w36) -> ("error out"=w29:errorcluster, "BME_DG_System out"=w30:refnum<class "BME_DG_System.lvclass">)  [unwired: 8 in]
  n44 = call "Activate All.vi"("error in (no error)"=w29, "BME_DG_System in"=w30) -> ("error out"=w26:errorcluster, "BME_DG_System out"=w28:refnum<class "BME_DG_System.lvclass">)  [unwired: 8 in]
  n45 = local read "ChnlParameter"() -> (w47:T5)
  n46 = call "ResetModuloCounters.vi"("error in (no error)"=w26, "Enum"=enum16{"Slaves only", "Slaves & Master"}."Slaves & Master", "BME_DG_System in"=w28) -> ("error out"=w25:errorcluster, "BME_DG_System out"=w27:refnum<class "BME_DG_System.lvclass">)  [unwired: 7 in]
  n47 = Obtain Queue(max queue size (-1, unlimited)=1, name (unnamed)="DGSysRef", element data type=w27) -> (queue out=w55:refnum<queue>, error out=w53:errorcluster)  [unwired: 2 in, 1 out]
  n48 = Obtain Queue(name (unnamed)="ChnlUpdateTasks", element data type=w47) -> (queue out=w48:refnum<queue>, error out=w49:errorcluster)  [unwired: 3 in, 1 out]
  n49 = Flush Queue(queue=w55, error in (no error)=w53) -> (queue out=w54:refnum<queue>, error out=w52:errorcluster)  [unwired: 1 out]
  n50 = Flush Queue(queue=w48, error in (no error)=w49) -> (queue out=w44:refnum<queue>, error out=w43:errorcluster)  [unwired: 1 out]
  n51 = Enqueue Element(queue=w54, element=w27, error in (no error)=w52) -> (queue out=w34:refnum<queue>, error out=w33:errorcluster)  [unwired: 1 in, 1 out]
  n52 = while {
    shift-right: [w164] -> _
    shift-left: w25 -> [w166]
    shift-right: [w162] -> w58
    shift-left: w33 -> [w163]
    tunnel: w34 -> [w167]
    tunnel: [w165] -> w60
    tunnel: w44 -> [w161]
    tunnel: w47 -> [w160]
    tunnel: [w158] -> w46
    shift-right: [w157] -> w42
    shift-left: w43 -> [w159]
    stop <- w168 stop-if-true
    n53 = event shown="[3] \"Update Delay formula\": Mouse Down" {
      selector: _ -> [_ _ _ _ _ _ _ _ _ _]
      dyn-events: _ -> [_ _ _ _ _ _ _ _ _ _]
      timeout: _ -> [_ _ _ _ _ _ _ _ _ _]
      tunnel: [_ w174 _ _ _ _ _ _ _ _] -> w168
      tunnel: w167 -> [w173 w183 w191 w216 w246 w258 w309 w328 w337 w383]
      tunnel: w166 -> [w172 w186 w192 w208 w237 w267 w314 w318 w345 w382]
      tunnel: [w173 w179 w191 w212 w242 w256 w307 w323 w331 w383] -> w165
      tunnel: [w172 w185 w187 w196 w226 w251 w314 w319 w338 w382] -> w164
      tunnel: w163 -> [w171 w182 w190 w215 w245 w257 w308 w326 w336 w379]
      tunnel: [w171 w180 w190 w213 w243 w255 w306 w324 w330 w379] -> w162
      tunnel: w161 -> [w170 w176 w189 w211 _ _ _ _ _ w374]
      tunnel: w160 -> [_ _ _ _ _ _ _ _ _ w378]
      tunnel: w159 -> [w169 w175 w188 w210 w241 w249 w313 w322 w329 w372]
      tunnel: [w170 w176 w189 w211 _ _ _ _ _ w371] -> w158
      tunnel: [w169 w175 w188 w210 w241 w249 w313 w322 w329 w370] -> w157
      event #0 {
        n54 = event-data() -> ()  [unwired: 1 in, 2 out]
      }
      event #1 {
        w174 = TRUE
        n55 = event-data() -> ()  [unwired: 1 in, 1 out]
        n56 = Dequeue Element(queue=w183, error in (no error)=w182) -> (queue out=w184:refnum<queue>, element=w177:refnum<class "BME_DG_System.lvclass">, error out=w181:errorcluster)  [unwired: 1 in, 1 out]
        n57 = call "Deactivate All.vi"("error in (no error)"=w186, "BME_DG_System in"=w177) -> ("error out"=w185:errorcluster, "BME_DG_System out"=w178:refnum<class "BME_DG_System.lvclass">)  [unwired: 8 in]
        n58 = local write "stop 2"(w174) -> ()
        n59 = Enqueue Element(queue=w184, element=w178, error in (no error)=w181) -> (queue out=w179:refnum<queue>, error out=w180:errorcluster)  [unwired: 1 in, 1 out]
        n60 = local write "stop 3"(w174) -> ()
      }
      event #2 {
        n61 = event-data() -> ()  [unwired: 1 in, 2 out]
        n62 = call <vilib>:"Clear Errors.vi"("error in (no error)"=w192) -> ("error out"=w187:errorcluster)  [unwired: 6 in]
      }
      event #3 {
        n63 = event-data() -> ()  [unwired: 1 in, 2 out]
        n64 = property on="Selected Chnl" class="Ring (strict)"() -> ("Strings []"=w206:string[], "Value"=w207:u16)  [unwired: 2 in, 2 out]
        n65 = Dequeue Element(queue=w216, error in (no error)=w215) -> (queue out=w217:refnum<queue>, element=w209:refnum<class "BME_DG_System.lvclass">, error out=w214:errorcluster)  [unwired: 1 in, 1 out]
        n66 = Index Array(array=w206, index=w207) -> (element=w195:string)
        n67 = call "Check new DelayFormula and Update Delays.vi"("error in (no error)"=w208, "Delay Formula"="DelayFormula", "ChnlName"=w195, "BME_DG_System in"=w209) -> ("error out"=w198:errorcluster, "Problem Chnls out"=→"Problem Chnls out":string[], "BME_DG_System out"=w200:refnum<class "BME_DG_System.lvclass">)  [unwired: 5 in]
        n68 = call "Get Chnl by Name.vi"("BME_DG_System in"=w200, "Chnl Name"=w195, "error in (no error)"=w198) -> ("BME_DG_System out"=w199:refnum<class "BME_DG_System.lvclass">, "Owner DG"=w201:refnum<class "BME_DG_Base.lvclass">, "error out"=w197:errorcluster)  [unwired: 7 in, 3 out]
        n69 = call-dynamic "Read objChnls.vi"("error in (no error)"=w197, "BME_DG_Base in"=w201) -> ("error out"=w202:errorcluster, "objChnls"=w204:refnum<class "BME_DG_Chnl.lvclass">[])  [unwired: 6 in, 2 out]
        n70 = for {
          tunnel: w204 -> [w224] mode=indexing
          tunnel: [w225] -> w203 mode=indexing
          shift-right: [w219] -> w196
          shift-left: w202 -> [w222]
          tunnel: [w218] -> w194 mode=indexing
          n71 = call-dynamic "Read TriggerModulo.vi"("error in (no error)"=w222, "BME_DG_Chnl in"=w224) -> ("error out"=w221:errorcluster, "BME_DG_Chnl out"=w223:refnum<class "BME_DG_Chnl.lvclass">)  [unwired: 7 in, 1 out]
          n72 = call-dynamic "Read ChnParameter.vi"("error in (no error)"=w221, "BME_DG_Chnl in"=w223) -> ("error out"=w219:errorcluster, "ChnParemater"=w225:T4, "BME_DG_Chnl out"=w220:refnum<class "BME_DG_Chnl.lvclass">)  [unwired: 4 in, 3 out]
          n73 = call-dynamic "Read DelayFormula.vi"("error in (no error)"=w219, "BME_DG_Chnl in"=w220) -> ("DelayFormula"=w218:string)  [unwired: 7 in, 2 out]
        }
        "DelayFormulas" <- w194
        n74 = local write "Chnls"(w203) -> ()
        n75 = Enqueue Element(queue=w217, element=w199, error in (no error)=w214) -> (queue out=w212:refnum<queue>, error out=w213:errorcluster)  [unwired: 1 in, 1 out]
      }
      event #4 {
        n76 = event-data() -> ()  [unwired: 1 in, 1 out]
        n77 = Dequeue Element(queue=w246, error in (no error)=w245) -> (queue out=w247:refnum<queue>, element=w238:refnum<class "BME_DG_System.lvclass">, error out=w244:errorcluster)  [unwired: 1 in, 1 out]
        n78 = property on="Selected Chnl" class="Ring (strict)"() -> ("Strings []"=w239:string[], "Value"=w240:u16)  [unwired: 2 in, 2 out]
        n79 = Index Array(array=w239, index=w240) -> (element=w236:string)
        n80 = call "Get Chnl by Name.vi"("BME_DG_System in"=w238, "Chnl Name"=w236, "error in (no error)"=w237) -> ("BME_DG_System out"=w232:refnum<class "BME_DG_System.lvclass">, "BME_DG_Chnl"=w235:refnum<class "BME_DG_Chnl.lvclass">, "error out"=w233:errorcluster)  [unwired: 7 in, 3 out]
        n81 = local read "ChnParam2write"() -> (w234:T4)
        n82 = call-dynamic "Write ChnParameter.vi"("error in (no error)"=w233, "ChnParemater"=w234, "BME_DG_Chnl in"=w235) -> ("error out"=w229:errorcluster, "BME_DG_Chnl out"=w230:refnum<class "BME_DG_Chnl.lvclass">)  [unwired: 7 in]
        n83 = call-dynamic "ModifyChnlHW.vi"("error in (no error)"=w229, "BME_DG_Chnl in"=w230) -> ("error out"=w227:errorcluster, "BME_DG_Chnl out"=w228:refnum<class "BME_DG_Chnl.lvclass">)  [unwired: 8 in]
        n84 = call "Write Chnl.vi"("error in (no error)"=w227, "BME_DG_Chnl.lvclass"=w228, "BME_DG_System in"=w232) -> ("error out"=w226:errorcluster, "BME_DG_System out"=w231:refnum<class "BME_DG_System.lvclass">)  [unwired: 7 in]
        n85 = Enqueue Element(queue=w247, element=w231, error in (no error)=w244) -> (queue out=w242:refnum<queue>, error out=w243:errorcluster)  [unwired: 1 in, 1 out]
      }
      event #5 {
        n86 = event-data() -> ("NewVal"=w269:u16)  [unwired: 1 in]
        n87 = property on="Selected Card" class="Ring (strict)"() -> ("Strings []"=w270:string[])  [unwired: 2 in, 2 out]
        n88 = Dequeue Element(queue=w258, error in (no error)=w257) -> (queue out=w259:refnum<queue>, element=w254:refnum<class "BME_DG_System.lvclass">, error out=w260:errorcluster)  [unwired: 1 in, 1 out]
        n89 = Index Array(array=w270, index=w269) -> (element=w268:string)
        n90 = call "Get DG by LogicalName.vi"("error in (no error)"=w267, "LogicalName"=w268, "BME_DG_System in"=w254) -> ("error out"=w252:errorcluster, "found?"=w266:bool, "BME_DG_Base.lvclass"=w265:refnum<class "BME_DG_Base.lvclass">, "BME_DG_System out"=w253:refnum<class "BME_DG_System.lvclass">)  [unwired: 5 in]
        n91 = property on="Selected Chnl" class="Ring (strict)"() -> ("Value"=w248:u16)  [unwired: 2 in, 2 out]
        n92 = case shown="True" w266 {
          tunnel: w265 -> [_ w280]
          tunnel: [_ w287] -> w264
          tunnel: [_ w286] -> w262
          tunnel: [_ w285] -> w263
          tunnel: [_ w281] -> w261
          tunnel: w252 -> [w272 w277]
          tunnel: [w271 w275] -> w250
          frame #0 {
            n93 = Build Array(w272) -> (w271:errorcluster[])
          }
          frame #1 {
            n94 = call-dynamic "Read IsActive.vi"("error in (no error)"=w277, "BME_DG_Base in"=w280) -> ("error out"=w278:errorcluster, "Active?"=w273:bool, "BME_DG_Base out"=w279:refnum<class "BME_DG_Base.lvclass">)  [unwired: 7 in]
            n95 = call-dynamic "Read Master.vi"("error in (no error)"=w278, "BME_DG_Base in"=w279) -> ("error out"=w282:errorcluster, "TriggerSettings"=w285:T2, "BME_DG_Base out"=w283:refnum<class "BME_DG_Base.lvclass">)  [unwired: 6 in, 1 out]
            n96 = property on="Activate" class="Bool (strict)"("DisabledEnum"=T9."Enabled" ("Disabled"), "Value"=w273) -> ()  [unwired: 2 in, 2 out]
            n97 = call-dynamic "Read objChnls.vi"("error in (no error)"=w282, "BME_DG_Base in"=w283) -> ("error out"=w276:errorcluster, "objChnls"=w284:refnum<class "BME_DG_Chnl.lvclass">[])  [unwired: 6 in, 2 out]
            n98 = for {
              tunnel: w284 -> [w293] mode=indexing
              tunnel: [w295] -> w287 mode=indexing
              tunnel: [w294] -> w286 mode=indexing
              tunnel: [w288] -> w281 mode=indexing
              tunnel: w276 -> [w291]
              tunnel: [w289] -> w275 mode=indexing
              n99 = call-dynamic "Read TriggerModulo.vi"("error in (no error)"=w291, "BME_DG_Chnl in"=w293) -> ("error out"=w290:errorcluster, "TriggerModulo"=w288:i32, "BME_DG_Chnl out"=w292:refnum<class "BME_DG_Chnl.lvclass">)  [unwired: 7 in]
              n100 = call-dynamic "Read ChnParameter.vi"("error in (no error)"=w290, "BME_DG_Chnl in"=w292) -> ("error out"=w289:errorcluster, "ChnParemater"=w294:T4, "Name"=w295:string)  [unwired: 4 in, 3 out]
            }
          }
        }
        "Chnls" <- w262
        "Modulo Settings" <- w261
        n101 = property on="Selected Chnl" class="Ring (strict)"("Val(Sgnl)"=w248) -> ()  [unwired: 2 in, 2 out]
        n102 = property on="Selected Chnl" class="Ring (strict)"("Strings []"=w264) -> ()  [unwired: 2 in, 2 out]
        n103 = local write "Trigger Base"(w263) -> ()
        n104 = Enqueue Element(queue=w259, element=w253, error in (no error)=w260) -> (queue out=w256:refnum<queue>, error out=w255:errorcluster)  [unwired: 1 in, 1 out]
        n105 = call <vilib>:"Merge Errors.vi"("error array in"=w250) -> ("error out"=w251:errorcluster)  [unwired: 6 in]
      }
      event #6 {
        n106 = event-data() -> ("NewVal"=w311:u16)  [unwired: 1 in]
        n107 = property on="Selected Chnl" class="Ring (strict)"() -> ("Strings []"=w312:string[])  [unwired: 2 in, 2 out]
        n108 = Index Array(array=w312, index=w311) -> (element=w301:string)
        n109 = Dequeue Element(queue=w309, error in (no error)=w308) -> (queue out=w310:refnum<queue>, element=w302:refnum<class "BME_DG_System.lvclass">, error out=w304:errorcluster)  [unwired: 1 in, 1 out]
        n110 = call "Get Chnl by Name.vi"("BME_DG_System in"=w302, "Chnl Name"=w301, "error in (no error)"=w304) -> ("BME_DG_System out"=w305:refnum<class "BME_DG_System.lvclass">, "BME_DG_Chnl"=w299:refnum<class "BME_DG_Chnl.lvclass">, "Owner DG"=w298:refnum<class "BME_DG_Base.lvclass">, "error out"=w303:errorcluster)  [unwired: 7 in, 2 out]
        n111 = call-dynamic "Read objChnls.vi"("BME_DG_Base in"=w298) -> ("objChnls"=w297:refnum<class "BME_DG_Chnl.lvclass">[])  [unwired: 7 in, 3 out]
        n112 = for {
          tunnel: w297 -> [w316] mode=indexing
          tunnel: [w315] -> w296 mode=indexing
          n113 = call-dynamic "Read DelayFormula.vi"("BME_DG_Chnl in"=w316) -> ("DelayFormula"=w315:string)  [unwired: 8 in, 2 out]
        }
        n114 = call-dynamic "Read DelayFormula.vi"("BME_DG_Chnl in"=w299) -> ("DelayFormula"=w300:string)  [unwired: 8 in, 2 out]
        n115 = local write "DelayFormulas"(w296) -> ()
        n116 = local write "DelayFormula"(w300) -> ()
        n117 = Enqueue Element(queue=w310, element=w305, error in (no error)=w303) -> (queue out=w307:refnum<queue>, error out=w306:errorcluster)  [unwired: 1 in, 1 out]
      }
      event #7 {
        n118 = event-data() -> ()  [unwired: 1 in, 1 out]
        n119 = Dequeue Element(queue=w328, error in (no error)=w326) -> (queue out=w327:refnum<queue>, element=w321:refnum<class "BME_DG_System.lvclass">, error out=w325:errorcluster)  [unwired: 1 in, 1 out]
        n120 = call "ResetModuloCounters.vi"("error in (no error)"=w318, "Enum"=enum16{"Slaves only", "Slaves & Master"}."Slaves & Master", "BME_DG_System in"=w321) -> ("error out"=w319:errorcluster, "BME_DG_System out"=w320:refnum<class "BME_DG_System.lvclass">)  [unwired: 7 in]
        n121 = Enqueue Element(queue=w327, element=w320, error in (no error)=w325) -> (queue out=w323:refnum<queue>, error out=w324:errorcluster)  [unwired: 1 in, 1 out]
      }
      event #8 {
        n122 = event-data() -> ()  [unwired: 1 in, 1 out]
        n123 = property on="Selected Card" class="Ring (strict)"() -> ("Strings []"=w348:string[], "Value"=w347:u16)  [unwired: 2 in, 2 out]
        n124 = Dequeue Element(queue=w337, error in (no error)=w336) -> (queue out=w334:refnum<queue>, element=w335:refnum<class "BME_DG_System.lvclass">, error out=w333:errorcluster)  [unwired: 1 in, 1 out]
        n125 = Index Array(array=w348, index=w347) -> (element=w346:string)
        n126 = call "Get DG by LogicalName.vi"("error in (no error)"=w345, "LogicalName"=w346, "BME_DG_System in"=w335) -> ("error out"=w343:errorcluster, "found?"=w339:bool, "BME_DG_Base.lvclass"=w344:refnum<class "BME_DG_Base.lvclass">, "BME_DG_System out"=w340:refnum<class "BME_DG_System.lvclass">)  [unwired: 5 in]
        n127 = case shown="True" w339 {
          tunnel: w344 -> [w352 w359]
          tunnel: w343 -> [w351 w357]
          tunnel: [w351 w361] -> w342
          tunnel: [w352 w360] -> w341
          frame #0 {
            n128 = property on="Activate" class="Bool (strict)"("Value"=FALSE ("Activate"), "DisabledEnum"=T9."Disabled and Grayed Out" ("Disabled")) -> ()  [unwired: 2 in, 2 out]
          }
          frame #1 {
            n129 = call-dynamic "Read IsActive.vi"("error in (no error)"=w357, "BME_DG_Base in"=w359) -> ("error out"=w356:errorcluster, "Active?"=w355:bool, "BME_DG_Base out"=w358:refnum<class "BME_DG_Base.lvclass">)  [unwired: 7 in]
            n130 = Not(x=w355) -> (.not. x?=w353:bool)
            n131 = case shown="True" w355 {
              tunnel: [w365 w367] -> w361
              tunnel: [w364 w368] -> w360
              tunnel: w358 -> [w363 w369]
              tunnel: w356 -> [w362 w366]
              frame #0 {
                n132 = call-dynamic "Activate.vi"("error in (no error)"=w362, "BME_DG_Base in"=w363) -> ("error out"=w365:errorcluster, "BME_DG_Base out"=w364:refnum<class "BME_DG_Base.lvclass">)  [unwired: 8 in]
              }
              frame #1 {
                n133 = call-dynamic "Deactivate.vi"("error in (no error)"=w366, "BME_DG_Base in"=w369) -> ("error out"=w367:errorcluster, "BME_DG_Base out"=w368:refnum<class "BME_DG_Base.lvclass">)  [unwired: 8 in]
              }
            }
            n134 = property on="Activate" class="Bool (strict)"("Value"=w353, "DisabledEnum"=T9."Enabled" ("Disabled")) -> ()  [unwired: 2 in, 2 out]
          }
        }
        n135 = call "Write DG.vi"("error in (no error)"=w342, "BME_DG_Base"=w341, "BME_DG_System in"=w340) -> ("error out"=w338:errorcluster, "BME_DG_System out"=w332:refnum<class "BME_DG_System.lvclass">)  [unwired: 7 in]
        n136 = Enqueue Element(queue=w334, element=w332, error in (no error)=w333) -> (queue out=w331:refnum<queue>, error out=w330:errorcluster)  [unwired: 1 in, 1 out]
      }
      event #9 {
        n137 = event-data() -> ()  [unwired: 1 in, 1 out]
        n138 = property on="Selected Chnl" class="Ring (strict)"() -> ("Strings []"=w380:string[], "Value"=w381:u16)  [unwired: 2 in, 2 out]
        n139 = Index Array(array=w380, index=w381) -> (element=w377:string)
        n140 = local read "ChnParam2write"() -> (w376:T4)
        n141 = local read "TriggerModulo"() -> (w375:u32)
        n142 = Bundle By Name(cluster=w378, "ChnlName"=w377, "ChnParam2write"=w376, "TriggerModulo"=w375) -> (w373:T5)
        n143 = Enqueue Element(queue=w374, element=w373, error in (no error)=w372) -> (queue out=w371:refnum<queue>, error out=w370:errorcluster)  [unwired: 1 in, 1 out]
      }
    }
    "error out" <- w166
  }
  n144 = while {
    tunnel: w34 -> [w391]
    shift-right: [w389] -> w57
    shift-left: w33 -> [w390]
    shift-right: [w386] -> w41
    shift-left: w25 -> [w388]
    tunnel: w44 -> [w385]
    tunnel: w43 -> [w384]
    stop <- w393 stop-if-true
    n145 = case shown="True" "ReadStatus" {
      tunnel: w391 -> [_ w422]
      tunnel: w390 -> [w396 w421]
      tunnel: [w396 w420] -> w389
      tunnel: w388 -> [w395 w418]
      tunnel: [w395 w404] -> w386
      tunnel: w385 -> [_ w408]
      tunnel: w384 -> [_ w407]
      frame #0 {
        n146 = Wait Until Next ms Multiple(millisecond multiple=u32 200) -> ()  [unwired: 1 out]
      }
      frame #1 {
        n147 = Dequeue Element(queue=w422, error in (no error)=w421) -> (queue out=w423:refnum<queue>, element=w419:refnum<class "BME_DG_System.lvclass">, error out=w424:errorcluster)  [unwired: 1 in, 1 out]
        n148 = Wait Until Next ms Multiple(millisecond multiple=u32 10) -> ()  [unwired: 1 out]
        n149 = call "ReadHWState.vi"("error in (no error)"=w418, "BME_DG_System in"=w419) -> ("error out"=w417:errorcluster, "Interrupts"=w413:u32[], "BME_DG_System out"=w416:refnum<class "BME_DG_System.lvclass">)  [unwired: 7 in]
        n150 = Or(x=u32 8192, y=w413) -> (x .or. y?=→"Interrupts":u32[])
        n151 = call "Read TriggersTillShot.vi"("error in (no error)"=w417, "BME_DG_System in"=w416) -> ("error out"=w409:errorcluster, "TriggerCounters"=→"TriggerCounters":i32[], "RemainingTriggers"=w415:T6, "BME_DG_System out"=w410:refnum<class "BME_DG_System.lvclass">)  [unwired: 6 in]
        n152 = call "CountsTillNextCommonTrigger.vi"("error in (no error)"=w409, "BME_DG_System in"=w410) -> ("error out"=w406:errorcluster, "LeastCommonMult"=w401:i32, "CountsRemains"=w402:i32, "BME_DG_System out"=w405:refnum<class "BME_DG_System.lvclass">)  [unwired: 6 in]
        "CountsRemains" <- w402
        n153 = Transpose 2D Array(2D array=w415) -> (transposed array=→"RemainingTriggers":T6)
        n154 = Equal?(x=w402, y=w401) -> (x = y?=w400:bool)
        n155 = case shown="No Error" w406 {
          selector: w406 -> [w428 w441]
          tunnel: w408 -> [w431 _]
          tunnel: w407 -> [w430 _]
          tunnel: w405 -> [w429 w442]
          tunnel: [w427 w441] -> w404
          tunnel: [w426 w442] -> w403
          tunnel: w400 -> [w425 _]
          frame #0 {
            n156 = case shown="True" w425 {
              tunnel: w431 -> [_ w440]
              tunnel: w430 -> [_ w439]
              tunnel: w429 -> [w433 w438]
              tunnel: w428 -> [w432 w436]
              tunnel: [w432 w435] -> w427
              tunnel: [w433 w434] -> w426
              frame #0 {
              }
              frame #1 {
                n157 = Flush Queue(queue=w440, error in (no error)=w439) -> (remaining elements=w437:T10)  [unwired: 2 out]
                n158 = call "Update Chnls.vi"("error in (no error)"=w436, "ChnlSettings"=w437, "BME_DG_System in"=w438) -> ("error out"=w435:errorcluster, "BME_DG_System out"=w434:refnum<class "BME_DG_System.lvclass">)  [unwired: 7 in]
              }
            }
          }
          frame #1 {
          }
        }
        n159 = Enqueue Element(queue=w423, element=w403, error in (no error)=w424) -> (error out=w420:errorcluster)  [unwired: 1 in, 2 out]
      }
    }
    n160 = Unbundle By Name(w386) -> ("status"=w392:bool)
    n161 = Or(x=w392, y="stop 2") -> (x .or. y?=w393:bool)
  }
  n162 = while {
    tunnel: w34 -> [w447]
    shift-right: [w444] -> w31
    shift-left: w33 -> [w446]
    stop <- w449 stop-if-true
    n163 = case shown="True" "Aknowledge interrupts" {
      tunnel: w447 -> [_ w459]
      tunnel: w446 -> [w451 w458]
      tunnel: [w451 w457] -> w444
      frame #0 {
      }
      frame #1 {
        n164 = Dequeue Element(queue=w459, error in (no error)=w458) -> (queue out=w456:refnum<queue>, element=w455:refnum<class "BME_DG_System.lvclass">, error out=w454:errorcluster)  [unwired: 1 in, 1 out]
        n165 = call "AcknowledgeInterrupts.vi"("error in (no error)"=w454, "BME_DG_System in"=w455) -> ("error out"=w452:errorcluster, "BME_DG_System out"=w453:refnum<class "BME_DG_System.lvclass">)  [unwired: 8 in]
        n166 = Enqueue Element(queue=w456, element=w453, error in (no error)=w452) -> (error out=w457:errorcluster)  [unwired: 1 in, 2 out]
      }
    }
    n167 = Wait Until Next ms Multiple(millisecond multiple=u32 500) -> ()  [unwired: 1 out]
    n168 = Unbundle By Name(w444) -> ("status"=w448:bool)
    n169 = Or(x=w448, y="stop 3") -> (x .or. y?=w449:bool)
  }
  n170 = call <vilib>:"Merge Errors.vi"("error in 3 (no error)"=w31, "error in 2 (no error)"=w57, "error in 1 (no error)"=w58) -> ("error out"=w59:errorcluster)  [unwired: 4 in]
  n171 = call <vilib>:"Merge Errors.vi"("error in 2 (no error)"=w41, "error in 1 (no error)"=w42) -> ("error out"=w40:errorcluster)  [unwired: 5 in]
  n172 = Release Queue(queue=w46, force destroy? (F)=TRUE, error in (no error)=w40) -> ()  [unwired: 3 out]
  n173 = Release Queue(queue=w60, error in (no error)=w59) -> ()  [unwired: 1 in, 3 out]
